vi "CRYCheck Value.vi"(8 "Data":T1={"Name"="", "Curve"=[], "X data"=1, "Y data"=1, "Z data"=1, "X axis"=0, "Y axis"=1, "Z axis"=1, "X unit"="Hz", "Y unit"="", "Z unit"="deg.", "X dB ref"=1.0, "Y dB ref"=1.0, "Z dB ref"=1.0, "single val"=FALSE, "protected"=FALSE, "display X"=TRUE, "display Y"=TRUE, "display Z"=TRUE, "Test Info"="", "Step No."=0, "Plot Settings"={"Color"=0, "Interpolation"=0, "Point Style"=0, "Line Style"=0, "Point Color"=0, "Line Width"=0, "Bar Plot Style"=0, "Fill To"=0}, "AutoProtect"=FALSE} {"Z data" items=["dB", "Lin"]; "X data" items=["dB", "Lin"]; "Y data" items=["dB", "Lin"]; "Z dB ref" format="%.1f"; "Z axis" items=["Log", "Lin"]; "X dB ref" format="%.1f"; "X axis" items=["Log", "Lin"]; "Y axis" items=["Log", "Lin"]; "Y dB ref" format="%.1f"; "Curve"."z" format="%.2f"; "Curve"."y" format="%.2f"; "Curve"."x" format="%.2f"}, 9 "Data Array":T2 {"Z data" items=["dB", "Lin"]; "X data" items=["dB", "Lin"]; "Y data" items=["dB", "Lin"]; "Z dB ref" format="%.1f"; "Z axis" items=["Log", "Lin"]; "X dB ref" format="%.1f"; "X axis" items=["Log", "Lin"]; "Y axis" items=["Log", "Lin"]; "Y dB ref" format="%.1f"; "Curve"."z" format="%.2f"; "Curve"."y" format="%.2f"; "Curve"."x" format="%.2f"}, 11 "Flatten Data Out":string) -> (3 "Single?":bool)   [LabVIEW 2013]
uses:
  CRYSystem/Typedef Control/CRYData Cluster Array.ctl
  CRYSystem/Typedef Control/CRYData Cluster.ctl
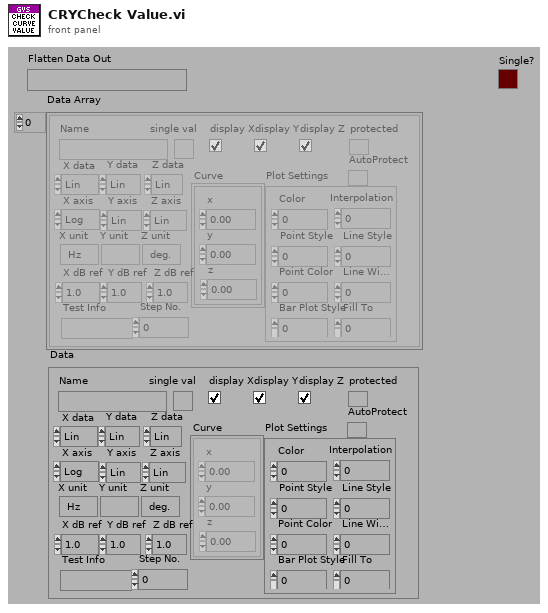
[diagram p1: front panel]
types:
  T1 = typedef "CRYData Cluster.ctl" = cluster{"Name":string, "Curve":cluster{"x":dbl, "y":dbl, "z":dbl}[], "X data":u16, "Y data":u16, "Z data":u16, "X axis":u16, "Y axis":u16, "Z axis":u16, "X unit":string, "Y unit":string, "Z unit":string, "X dB ref":dbl, "Y dB ref":dbl, "Z dB ref":dbl, "single val":bool, "protected":bool, "display X":bool, "display Y":bool, "display Z":bool, "Test Info":string, "Step No.":i32, "Plot Settings":cluster{"Color":u32, "Interpolation":u8, "Point Style":u8, "Line Style":u8, "Point Color":u32, "Line Width":u8, "Bar Plot Style":u8, "Fill To":i16}, "AutoProtect":bool}
  T2 = typedef "CRYData Cluster Array.ctl" = T1[]
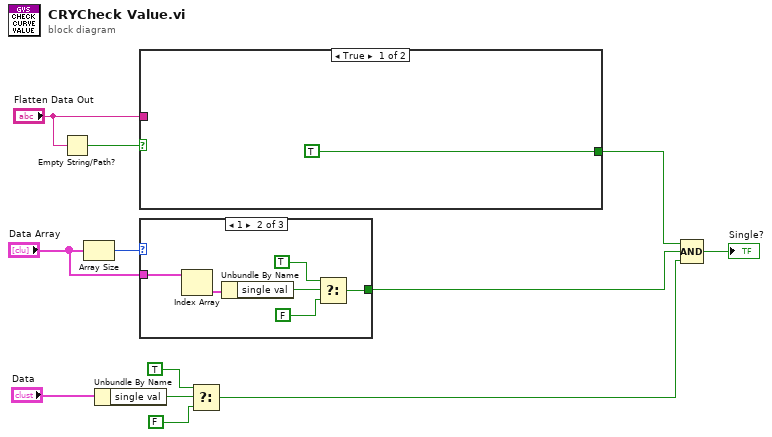
[diagram p0: block diagram]
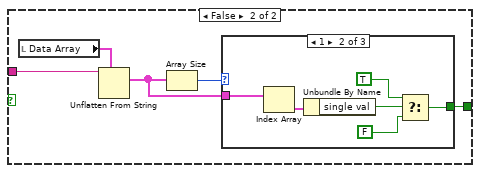
[diagram p2: hidden frame]
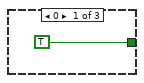
[diagram p3: hidden frame]
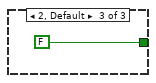
[diagram p4: hidden frame]
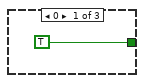
[diagram p5: hidden frame]
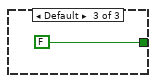
[diagram p6: hidden frame]
diagram:
  n1 = Empty String/Path?(string/path="Flatten Data Out") -> (empty?=w6:bool)
  n2 = Array Size(array="Data Array") -> (size(s)=w12:i32)
  n3 = Unbundle By Name("Data") -> ("single val"=w3:bool)
  n4 = case shown="True" w6 {
    tunnel: [TRUE w17] -> w9
    tunnel: "Flatten Data Out" -> [_ w14]
    frame True {
    }
    frame False {
      n5 = local read "Data Array"() -> (w16:T2)
      n6 = Unflatten From String(type=w16, binary string=w14) -> (value=w15:T2)  [unwired: 2 in, 3 out]
      n7 = Array Size(array=w15) -> (size(s)=w18:i32)
      n8 = case shown="1" w18 {
        tunnel: [TRUE w21 FALSE] -> w17
        tunnel: w15 -> [_ w20 _]
        frame 0 {
        }
        frame 1 {
          n9 = Index Array(array=w20) -> (element=w25:T1)  [unwired: 1 in]
          n10 = Unbundle By Name(w25) -> ("single val"=w24:bool)
          n11 = Select(t=TRUE, s=w24, f=FALSE) -> (s? t:f=w21:bool)
        }
        frame 2, Default {
        }
      }
    }
  }
  n12 = case shown="1" w12 {
    tunnel: "Data Array" -> [_ w33 _]
    tunnel: [TRUE w28 FALSE] -> w8
    frame 0 {
    }
    frame 1 {
      n13 = Index Array(array=w33) -> (element=w32:T1)  [unwired: 1 in]
      n14 = Unbundle By Name(w32) -> ("single val"=w31:bool)
      n15 = Select(t=TRUE, s=w31, f=FALSE) -> (s? t:f=w28:bool)
    }
    frame Default {
    }
  }
  n16 = Select(t=TRUE, s=w3, f=FALSE) -> (s? t:f=w1:bool)
  n17 = Compound Arithmetic op=AND(w9, w8, w1) -> (→"Single?":bool)
